vi "Queue Comms Dequeue.vi"(8 "Error In":errorcluster) -> (0 "Error Out":errorcluster, 2 "Message Data":T1)   [LabVIEW 2015, in "Controller.lvlib"]
doc: "VI used to dequeue data from queue."
uses:
  Controller.lvlib
  Private Controls/Module Data Cluster.ctl
  Private Controls/Module Action.ctl
  Private Controls/Queue FGV Action.ctl
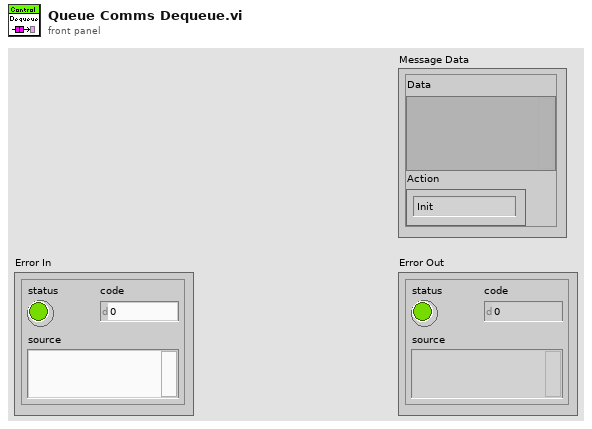
[diagram p1: front panel]
types:
  T1 = typedef "Controller.lvlib/Module Data Cluster.ctl" = cluster{"Data":variant, "Action":T2}
  T2 = typedef "Controller.lvlib/Module Action.ctl" = enum16{"Init", "Close", "Error", "Start Wash Operation"}
  T3 = typedef "Controller.lvlib/Queue FGV Action.ctl" = enum16{"Set", "Get", "Release"}
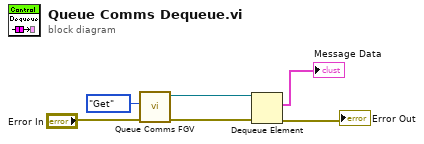
[diagram p0: block diagram]
diagram:
  n1 = call "Queue Comms FGV.vi"("Error In"="Error In", "Queue Option"=Queue_FGV_Action."Get") -> ("Error Out"=w6:errorcluster, "Out"=w5:refnum<queue>)  [unwired: 8 in]
  n2 = Dequeue Element(queue=w5, error in (no error)=w6) -> (element=→"Message Data":T1, error out=→"Error Out":errorcluster)  [unwired: 1 in, 2 out]
